vi "FPGA_Qudi_merFISH_trigger_camera_synchro_laser_lines_measure_QPD.vi"(3 "N Z positions":i32) -> ()   [LabVIEW 2015]
uses:
  <vilib>/Platform/TimedLoop/XDataNode/timing_clust.ctl
  <vilib>/Platform/TimedLoop/XDataNode/nitl_modes.ctl
  <vilib>/Platform/TimedLoop/XDataNode/wakeup.ctl
  <vilib>/rvi/FXPMathLib/basic elements/FxpIntAccumulator/subVIs/nifxpmath_IntAccumulator_SimConfig.ctl
  <vilib>/rvi/Emulation/niFpgaGetClockAttributes.vi
  <vilib>/rvi/Emulation/niFpgaSctlEmulationGetInTimedLoop.vi
  <vilib>/rvi/Emulation/niFpgaEmulationReportErrorSimple.vi
  <vilib>/rvi/eio/common/nirviEmuTemplateMethod_errors.vi
  <vilib>/rvi/Emulation/niFpgaProcessEmulError.vi
  <vilib>/rvi/Analysis/common/codeGenErrors/XNode/niFpgaXNodeCodeGenErrorHandle.vi
  <vilib>/rvi/Emulation/niFpgaCriticalErrorInLSC.vi
  <vilib>/rvi/FXPMathLib/basic elements/FxpIntAccumulator/simVIs/DllFxpIntAccumulator_sub.vi
  <vilib>/eio/EIONode/EIONode.xnode
  <vilib>/rvi/Analysis/measure/dc-rms/XNode/niFpgaDC-RMS.xnode
  <vilib>/Platform/TimedLoop/XDataNode/XDataNode.xnode
  <vilib>/rvi/FXPMathLib/basic elements/FxpIntAccumulator/XNode/nifxpmath_IntAccumulator.xnode
  <vilib>/Platform/TimedLoop/XDataNode/XDNodeRunTimeDep.lvlib
panel:
  out "n cycles":i32
  out "DIo1 2":i32
  out "DIo3":i32
  out "DIo1":i32
  in  "stop":bool
  out "duration (ms)":u32
  out "QPD":T1
  in  "Reset counter":bool
  out "Images acquired":i32
  in  "Laser lines":i32[](array[numeric])=[0, 0, 0, 0, 0]
  in  "Laser power":i16[](array[numeric])=[0, 0, 0, 0, 0]
  in  "N laser lines":i32
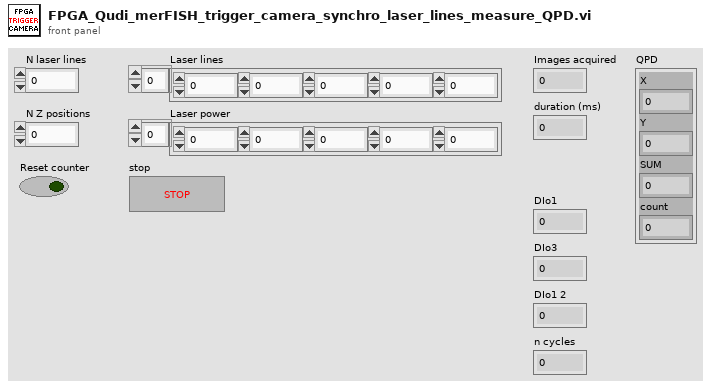
[diagram p1: front panel]
types:
  T1 = cluster{"X":sgl, "Y":sgl, "SUM":sgl, "count":u32}
  T2 = typedef "XDNodeRunTimeDep.lvlib/timing_clust.ctl" = cluster{"Expected End [f-1]":u64, "Actual End [f-1]":u64, "Finished Late? [f-1]":bool, "Expected End [i-1]":u64, "Actual End [i-1]":u64, "Finished Late? [i-1]":bool, "Expected Start [i]":u64, "Actual Start [i]":u64, "Expected Start [f]":u64, "Actual Start [f]":u64, "Source Name":string, "Structure Name":string, "Period":i64, "Deadline":i64, "Offset":i64, "Start":i64, "Priority":i32, "Timeout":i32, "Mode":T3, "Wakeup Reason":T4, "Error":errorcluster, "Source Type":string, "Secondary Source Type":string, "Global End Time":u64, "Global Start Time":u64, "Frame Duration":u64, "Iteration Duration":u64, "Assigned CPU":i32, "I/O Scan Engine Mode":u32}
  T3 = typedef "XDNodeRunTimeDep.lvlib/nitl_modes.ctl" = enum32{"No Change", "Process missed periods, maintain original phase", "Discard missed periods, maintain original phase", "Process missed periods, ignore original phase", "Discard missed periods, ignore original phase"}
  T4 = typedef "XDNodeRunTimeDep.lvlib/wakeup.ctl" = enum32{"Normal", "Aborted", "Asynchronous wakeup", "Timing source error", "Timed loop error", "Timeout"}
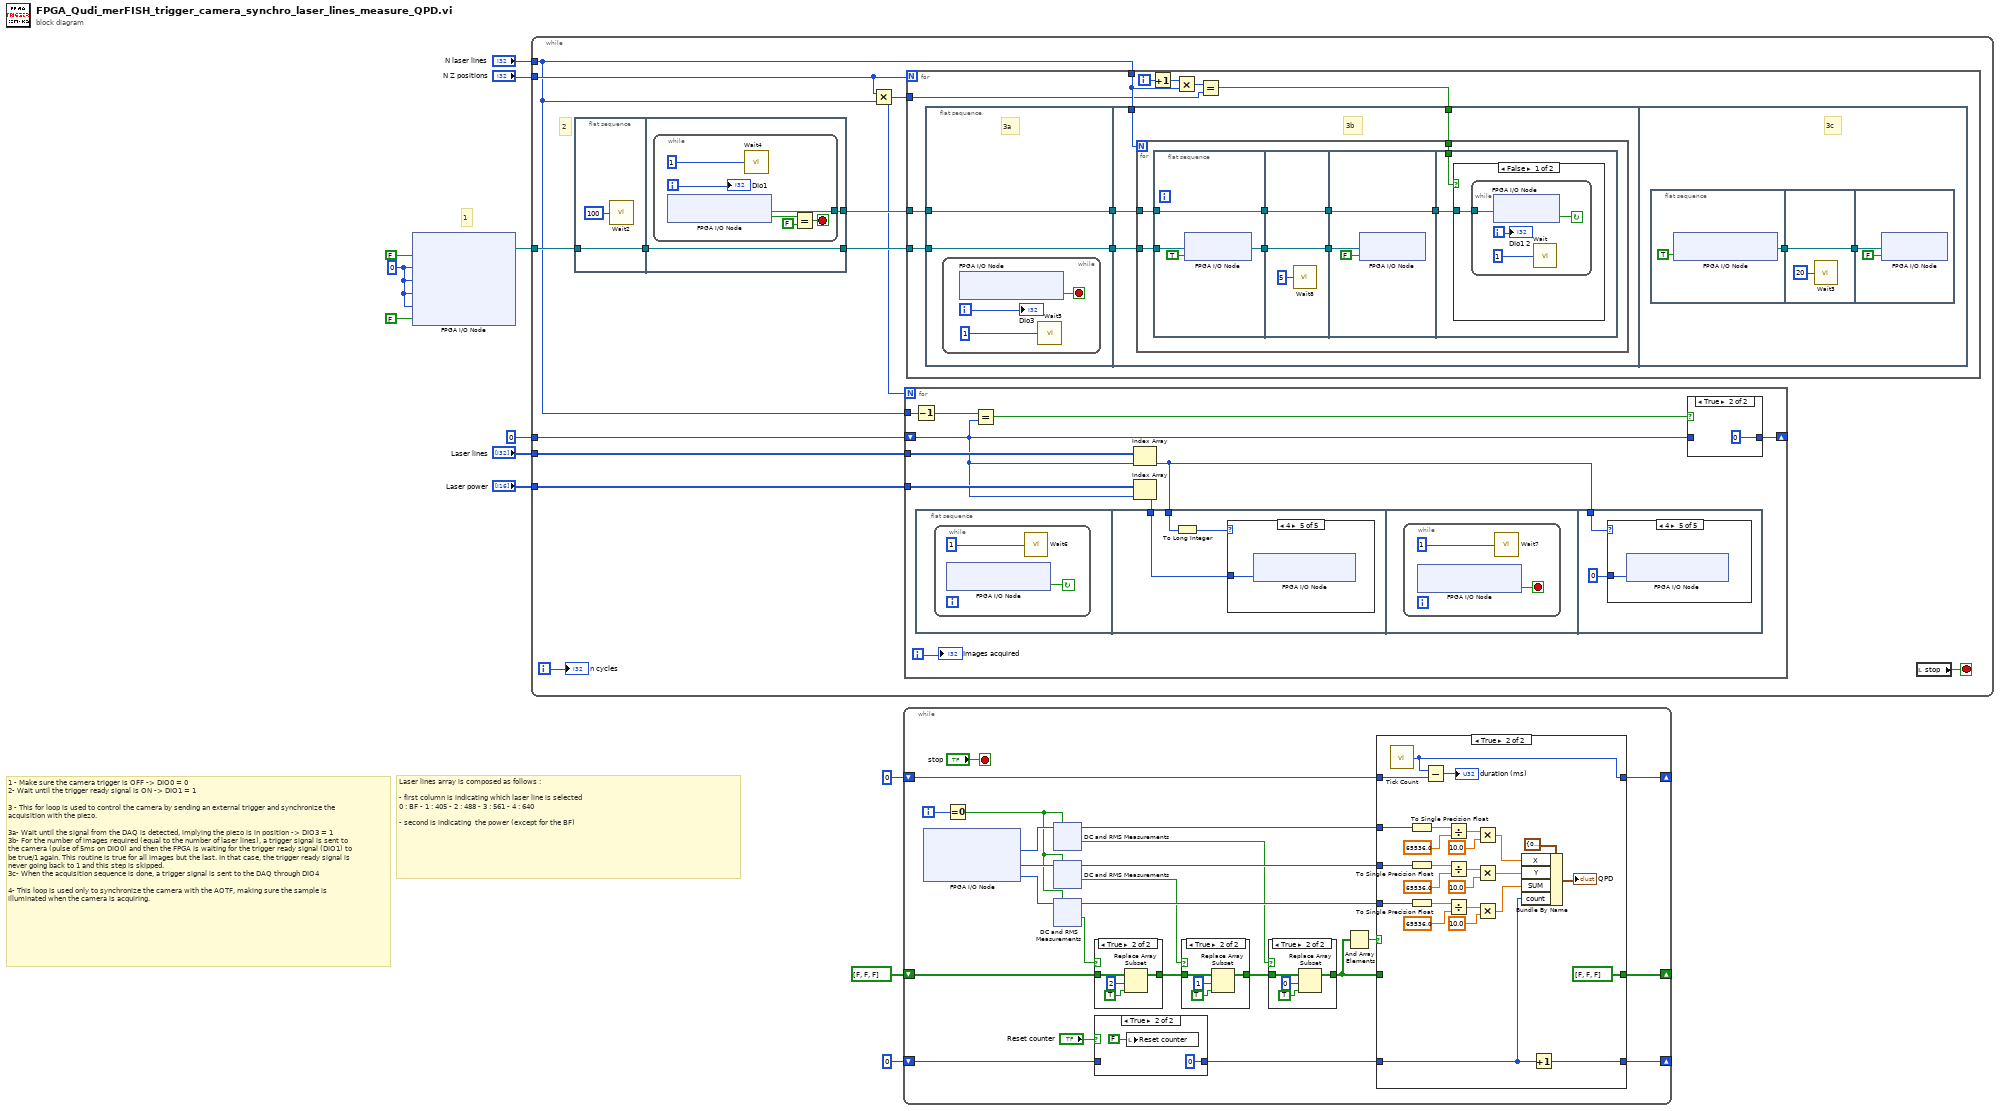
[diagram p0: block diagram]
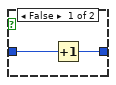
[diagram p2: hidden frame]
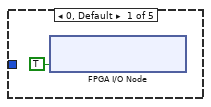
[diagram p3: hidden frame]
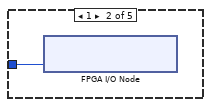
[diagram p4: hidden frame]
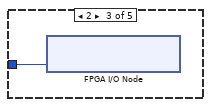
[diagram p5: hidden frame]
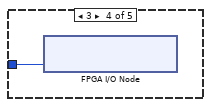
[diagram p6: hidden frame]
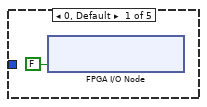
[diagram p7: hidden frame]
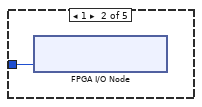
[diagram p8: hidden frame]
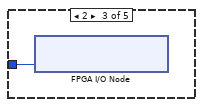
[diagram p9: hidden frame]
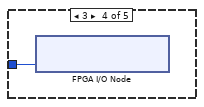
[diagram p10: hidden frame]
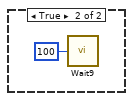
[diagram p11: hidden frame]
diagram:
  w5 = i16 0 ("Connector0/AO0")
  # "Laser lines array is composed as follows :\n\n- first column is indicating which laser line is selected \n0 : BF - 1 : 405 - 2 : 488 - 3 : 561 - 4 : 640\n\n- second is indicating  the power (except for the BF)"
  # "1"
  # "1 - Make sure the camera trigger is OFF -> DIO0 = 0\n2- Wait until the trigger ready signal is ON -> DIO1 = 1\n\n3 - This for loop is used to control the camera by sending an external trigger and synchronize the acquisition with the piezo.\n\n3a- Wait until the signal from the DAQ is detected, implying the piezo is in position -> DIO3 = 1 \n3b- For the number of images required (equal to the number of laser lines), a trigger signal is sent to the camera (pulse of 5ms on DIO0) and then the FPGA is waiting for the trigger ready signal (DIO1) to be true/1 again. This routine is true for all images but the last. In that case, the trigger ready signal is never going back to 1 and this step is skipped. \n3c- When the acquisition sequence is done, a trigger signal is sent to the DAQ through DIO4\n\n4- This loop is used only to synchronize the camera with the AOTF, making sure the sample is illuminated when the camera is acquiring."
  n1 = xnode "FPGA I/O Node"("Connector0/DIO0"=FALSE, "Connector0/AO0"=w5, "Connector0/AO1"=w5, "Connector0/AO2"=w5, "Connector0/AO3"=w5, "Connector0/DIO5"=FALSE) -> ("FPGA I/O Out"=w11:refnum<k21>)  [unwired: 6 in, 5 out]
  n2 = while {
    tunnel: w11 -> [w23]
    tunnel: "Laser power" -> [w20]
    tunnel: "Laser lines" -> [w19]
    tunnel: 0 -> [w18]
    tunnel: "N Z positions" -> [w17]
    tunnel: "N laser lines" -> [w16]
    i -> [w14]
    stop <- w15 stop-if-true
    # "2"
    n3 = flat-sequence {
      tunnel: w23 -> [w58]
      tunnel: [w58] -> w24
      tunnel: w24 -> [w60]
      tunnel: [w60] -> w22
      tunnel: [w59] -> w21
      frame #0 {
        n4 = call "Wait2"("Count(uSec)"=u32 100 ("Count(mSec)")) -> ()  [unwired: 1 out]
      }
      frame #1 {
        n5 = while {
          tunnel: [w66] -> w59
          i -> [w62]
          stop <- w63 stop-if-true
          n6 = xnode "FPGA I/O Node"() -> ("Connector0/DIO1"=w65:bool, "FPGA I/O Out"=w66:refnum<k21>)  [unwired: 1 in]
          n7 = call "Wait4"("Count(mSec)"=u32 1) -> ()  [unwired: 1 out]
          n8 = Equal?(x=w65, y=FALSE) -> (x = y?=w63:bool)
          "DIo1" <- w62
        }
      }
    }
    n9 = Multiply(x=w17, y=w16) -> (x*y=w13:i32)
    n10 = for {
      N: w13 -> [_]
      shift-right: [w32] -> _
      shift-left: w18 -> [w29]
      tunnel: w19 -> [w31]
      tunnel: w20 -> [w30]
      tunnel: w16 -> [w27]
      i -> [w25]
      n11 = Decrement(x=w27) -> (x-1=w26:i32)
      n12 = flat-sequence {
        tunnel: w34 -> [w41]
        tunnel: w28 -> [w40]
        tunnel: w34 -> [w50]
        frame #0 {
          n13 = while {
            stop <- w39 continue-if-true
            n14 = xnode "FPGA I/O Node"() -> ("Connector0/DIO2"=w39:bool)  [unwired: 1 in, 1 out]
            n15 = call "Wait6"("Count(mSec)"=u32 1) -> ()  [unwired: 1 out]
          }
        }
        frame #1 {
          n16 = To Long Integer(number=w41) -> (32bit integer=w42:i32)
          n17 = case shown="4" w42 {
            tunnel: w40 -> [_ w44 w45 w46 w47]
            frame 0, Default {
              n18 = xnode "FPGA I/O Node"("Connector0/DIO5"=TRUE) -> ()  [unwired: 1 in, 1 out]
            }
            frame 1 {
              n19 = xnode "FPGA I/O Node"("Connector0/AO2"=w44) -> ()  [unwired: 1 in, 1 out]
            }
            frame 2 {
              n20 = xnode "FPGA I/O Node"("Connector0/AO3"=w45) -> ()  [unwired: 1 in, 1 out]
            }
            frame 3 {
              n21 = xnode "FPGA I/O Node"("Connector0/AO0"=w46) -> ()  [unwired: 1 in, 1 out]
            }
            frame 4 {
              n22 = xnode "FPGA I/O Node"("Connector0/AO1"=w47) -> ()  [unwired: 1 in, 1 out]
            }
          }
        }
        frame #2 {
          n23 = while {
            stop <- w49 stop-if-true
            n24 = xnode "FPGA I/O Node"() -> ("Connector0/DIO2"=w49:bool)  [unwired: 1 in, 1 out]
            n25 = call "Wait7"("Count(mSec)"=u32 1) -> ()  [unwired: 1 out]
          }
        }
        frame #3 {
          n26 = case shown="4" w50 {
            tunnel: i16 0 -> [_ w53 w54 w55 w56]
            frame 0, Default {
              n27 = xnode "FPGA I/O Node"("Connector0/DIO5"=FALSE) -> ()  [unwired: 1 in, 1 out]
            }
            frame 1 {
              n28 = xnode "FPGA I/O Node"("Connector0/AO2"=w53) -> ()  [unwired: 1 in, 1 out]
            }
            frame 2 {
              n29 = xnode "FPGA I/O Node"("Connector0/AO3"=w54) -> ()  [unwired: 1 in, 1 out]
            }
            frame 3 {
              n30 = xnode "FPGA I/O Node"("Connector0/AO0"=w55) -> ()  [unwired: 1 in, 1 out]
            }
            frame 4 {
              n31 = xnode "FPGA I/O Node"("Connector0/AO1"=w56) -> ()  [unwired: 1 in, 1 out]
            }
          }
        }
      }
      n32 = Equal?(x=w26, y=w29) -> (x = y?=w33:bool)
      n33 = Index Array(array=w31, index=w29) -> (element=w34:i32)
      n34 = Index Array(array=w30, index=w29) -> (element=w28:i16)
      n35 = case shown="True" w33 {
        tunnel: w29 -> [w36 _]
        tunnel: [w35 0] -> w32
        frame False {
          n36 = Increment(x=w36) -> (x+1=w35:i32)
        }
        frame True {
        }
      }
      "Images acquired" <- w25
    }
    n37 = for {
      N: w17 -> [_]
      tunnel: w22 -> [w75]
      tunnel: w21 -> [w76]
      tunnel: w16 -> [w70]
      tunnel: w13 -> [w67]
      i -> [w72]
      n38 = flat-sequence {
        tunnel: w75 -> [w77]
        tunnel: w76 -> [w78]
        tunnel: [w78] -> w74
        tunnel: [w77] -> w73
        tunnel: w74 -> [w85]
        tunnel: w73 -> [w84]
        tunnel: w70 -> [w83]
        tunnel: w69 -> [w82]
        frame #0 {
          # "3a"
          n39 = while {
            i -> [w80]
            stop <- w81 stop-if-true
            n40 = xnode "FPGA I/O Node"() -> ("Connector0/DIO3"=w81:bool)  [unwired: 1 in, 1 out]
            n41 = call "Wait5"("Count(mSec)"=u32 1) -> ()  [unwired: 1 out]
            "DIo3" <- w80
          }
        }
        frame #1 {
          # "3b"
          n42 = for {
            N: w83 -> [_]
            tunnel: w85 -> [w88]
            tunnel: w84 -> [w87]
            tunnel: w82 -> [w86]
            n43 = flat-sequence {
              tunnel: [w96] -> w93
              tunnel: [w94] -> w92
              tunnel: w87 -> [w95]
              tunnel: w88 -> [w94]
              tunnel: w93 -> [w100]
              tunnel: [w100] -> w91
              tunnel: [w99] -> w90
              tunnel: w92 -> [w99]
              tunnel: w91 -> [w102]
              tunnel: [w101] -> w89
              tunnel: w90 -> [w101]
              tunnel: w89 -> [w105]
              tunnel: w86 -> [w104]
              frame #0 {
                n44 = xnode "FPGA I/O Node"("I/O Item"=TRUE ("Connector0/DIO0"), "FPGA I/O In"=w95) -> ("FPGA I/O Out"=w96:refnum<k21>)
              }
              frame #1 {
                n45 = call "Wait8"("Count(mSec)"=u32 5) -> ()  [unwired: 1 out]
              }
              frame #2 {
                n46 = xnode "FPGA I/O Node"("I/O Item"=FALSE ("Connector0/DIO0"), "FPGA I/O In"=w102) -> ()  [unwired: 1 out]
              }
              frame #3 {
                n47 = case shown="False" w104 {
                  tunnel: w105 -> [w106 _]
                  frame False {
                    n48 = while {
                      tunnel: w106 -> [w110]
                      i -> [w108]
                      stop <- w109 continue-if-true
                      n49 = xnode "FPGA I/O Node"("FPGA I/O In"=w110) -> ("I/O Item"=w109:bool)  [unwired: 1 out]
                      n50 = call "Wait"("Count(mSec)"=u32 1) -> ()  [unwired: 1 out]
                      "DIo1 2" <- w108
                    }
                  }
                  frame True {
                    n51 = call "Wait9"("Count(uSec)"=u32 100 ("Count(mSec)")) -> ()  [unwired: 1 out]
                  }
                }
              }
            }
          }
        }
        frame #2 {
          # "3c"
          n52 = flat-sequence {
            tunnel: [w115] -> w113
            tunnel: w113 -> [w116]
            tunnel: [w116] -> w112
            tunnel: w112 -> [w118]
            frame #0 {
              n53 = xnode "FPGA I/O Node"("Connector0/DIO4"=TRUE) -> ("FPGA I/O Out"=w115:refnum<k21>)  [unwired: 1 in]
            }
            frame #1 {
              n54 = call "Wait3"("Count(mSec)"=u32 20) -> ()  [unwired: 1 out]
            }
            frame #2 {
              n55 = xnode "FPGA I/O Node"("I/O Item"=FALSE ("Connector0/DIO0"), "FPGA I/O In"=w118) -> ()  [unwired: 1 out]
            }
          }
        }
      }
      n56 = Increment(x=w72) -> (x+1=w71:i32)
      n57 = Multiply(x=w71, y=w70) -> (x*y=w68:i32)
      n58 = Equal?(x=w68, y=w67) -> (x = y?=w69:bool)
    }
    n59 = local read "stop"() -> (w15:bool)
    "n cycles" <- w14
  }
  n60 = while {
    shift-right: [w126] -> _
    shift-left: bool[] [FALSE, FALSE, FALSE] ("initialized array") -> [w134]
    shift-right: [w124] -> _
    shift-left: u32 0 -> [w125]
    shift-right: [w123] -> _
    shift-left: u32 0 -> [w121]
    i -> [w141]
    stop <- "stop" stop-if-true
    n61 = xnode "FPGA I/O Node"() -> ("Connector0/AI0"=w143:i16, "Connector0/AI1"=w139:i16, "Connector0/AI2"=w138:i16)  [unwired: 3 in, 3 out]
    n62 = Equal To 0?(x=w141) -> (x = 0?=w135:bool)
    n63 = xnode "DC and RMS Measurements"("input data"=w143, "reset"=w135) -> ("DC"=w140:i16, "output valid"=w129:bool)
    n64 = xnode "DC and RMS Measurements"("input data"=w139, "reset"=w135) -> ("DC"=w137:i16, "output valid"=w130:bool)
    n65 = xnode "DC and RMS Measurements"("input data"=w138, "reset"=w135) -> ("DC"=w136:i16, "output valid"=w131:bool)
    n66 = case shown="True" w131 {
      tunnel: w134 -> [w152 w155]
      tunnel: [w152 w153] -> w133
      frame False {
      }
      frame True {
        n67 = Replace Array Subset(array=w155, new element=TRUE, index=2) -> (w153:bool[])
      }
    }
    n68 = case shown="True" "Reset counter" {
      tunnel: w121 -> [w144 _]
      tunnel: [w144 u32 0] -> w120
      frame False {
      }
      frame True {
        n69 = local write "Reset counter"(FALSE ("Reset counter")) -> ()
      }
    }
    n70 = case shown="True" w130 {
      tunnel: w133 -> [w157 w160]
      tunnel: [w157 w158] -> w132
      frame False {
      }
      frame True {
        n71 = Replace Array Subset(array=w160, new element=TRUE, index=1) -> (w158:bool[])
      }
    }
    n72 = case shown="True" w129 {
      tunnel: [w147 w149] -> w127
      tunnel: w132 -> [w147 w148]
      frame False {
      }
      frame True {
        n73 = Replace Array Subset(array=w148, new element=TRUE, index=0) -> (w149:bool[])
      }
    }
    n74 = And Array Elements(Boolean array=w127) -> (logical AND=w128:bool)
    n75 = case shown="True" w128 {
      tunnel: w140 -> [_ w190]
      tunnel: w137 -> [_ w181]
      tunnel: w136 -> [_ w176]
      tunnel: w127 -> [w164 _]
      tunnel: [w164 bool[] [FALSE, FALSE, FALSE] ("initialized array")] -> w126
      tunnel: w125 -> [w163 w171]
      tunnel: [w163 w169] -> w124
      tunnel: w120 -> [w162 w166]
      tunnel: [w162 w165] -> w123
      frame False {
      }
      frame True {
        n76 = call "Tick Count"() -> ("Tick Count(mSec)"=w169:u32)
        n77 = To Single Precision Float(number=w190) -> (single precision float=w189:sgl)
        n78 = To Single Precision Float(number=w181) -> (single precision float=w182:sgl)
        n79 = To Single Precision Float(number=w176) -> (single precision float=w180:sgl)
        n80 = Subtract(x=w169, y=w171) -> (x-y=→"duration (ms)":u32)
        n81 = Divide(x=w189, y=sgl 65536.0) -> (x/y=w187:sgl)
        n82 = Divide(x=w182, y=sgl 65536.0) -> (x/y=w184:sgl)
        n83 = Divide(x=w180, y=sgl 65536.0) -> (x/y=w178:sgl)
        n84 = Multiply(x=w187, y=sgl 10.0) -> (x*y=w175:sgl)
        n85 = Multiply(x=w184, y=sgl 10.0) -> (x*y=w174:sgl)
        n86 = Multiply(x=w178, y=sgl 10.0) -> (x*y=w173:sgl)
        n87 = Bundle By Name(cluster=T1 {"X"=0.0, "Y"=0.0, "SUM"=0.0, "count"=0} ("output cluster"), "X"=w175, "Y"=w174, "SUM"=w173, "count"=w166) -> (→"QPD":T1)
        n88 = Increment(x=w166) -> (x+1=w165:u32)
      }
    }
  }
